vi "NI.AI.vi"   [LabVIEW 2012, in "Lib_UEL.ATE.lvlib" / "Lib_PCI6221.lvlib"]
uses:
  Lib_PCI6221.lvlib
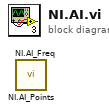
[diagram p0: block diagram]
diagram:
  n1 = call "NI.AI_Points.vi"() -> ()  [unwired: 9 in, 7 out]
  n2 = call "NI.AI_Freq.vi"() -> ()  [unwired: 5 in, 7 out]
